vi "20190420 Subvi AO trigger old.vi"(9 "Delay_ticks":u32, 11 "Trigger":bool) -> (1 "IteratorDirection":bool, 3 "Stop":bool)   [LabVIEW 2017]
uses:
  GV trigger external AODO.vi
  GV frame counter.vi
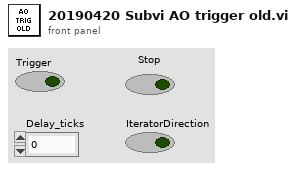
[diagram p1: front panel]
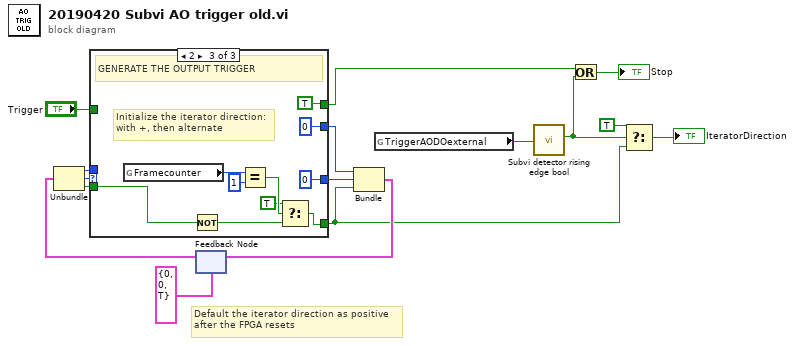
[diagram p0: block diagram]
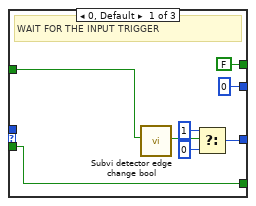
[diagram p2: hidden frame]
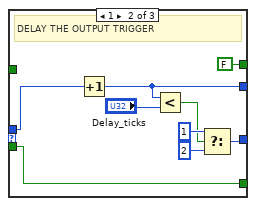
[diagram p3: hidden frame]
diagram:
  # "Default the iterator direction as positive\nafter the FPGA resets"
  n1 = feedback #1(cluster{u16, "f":u8, bool} {0, "f"=0, TRUE}) -> (w8:cluster{u32, "f":u8, bool})
  n2 = Unbundle(w8) -> (w9:u32, "f"=w11:u8, w12:bool)
  n3 = case shown="2" w11 {
    tunnel: [u32 0 w32 u32 0] -> w6
    tunnel: [w24 w28 u8 0 ("f")] -> w10
    tunnel: w9 -> [_ w33 _]
    tunnel: [FALSE FALSE TRUE] -> w2
    tunnel: [w19 w26 w34] -> w3
    tunnel: w12 -> [w19 w26 w36]
    tunnel: "Trigger" -> [w17 _ _]
    frame 0, Default {
      # "WAIT FOR THE INPUT TRIGGER"
      n4 = call "Subvi detector edge change bool.vi"("Input"=w17) -> ("Output"=w18:bool)  [unwired: 8 in]
      n5 = Select(t=u8 1, s=w18, f=u8 0) -> (s? t:f=w24:u8)
    }
    frame 1 {
      # "DELAY THE OUTPUT TRIGGER"
      n6 = Increment(x=w33) -> (x+1=w32:u32)
      n7 = Less?(x=w32, y="Delay_ticks") -> (x < y?=w30:bool)
      n8 = Select(t=u8 1, s=w30, f=u8 2) -> (s? t:f=w28:u8)
    }
    frame 2 {
      # "Initialize the iterator direction:\nwith +, then alternate"
      # "GENERATE THE OUTPUT TRIGGER"
      n9 = global read "GV frame counter.vi" "Framecounter"() -> (w38:i16)
      n10 = Not(x=w36) -> (.not. x?=w35:bool)
      n11 = Equal?(x=w38, y=i16 1) -> (x = y?=w40:bool)
      n12 = Select(t=TRUE, s=w40, f=w35) -> (s? t:f=w34:bool)
    }
  }
  n13 = Bundle(w6, "f"=w10, w3) -> (w7:cluster{u32, "f":u8, bool})  [unwired: 1 in]
  n14 = feedback-in #1(w7) -> ()
  n15 = global read "GV trigger external AODO.vi" "TriggerAODOexternal"() -> (w14:bool)
  n16 = call "Subvi detector rising edge bool.vi"("Input"=w14) -> ("Output"=w1:bool)  [unwired: 10 in]
  n17 = Or(x=w2, y=w1) -> (x .or. y?=→"Stop":bool)
  n18 = Select(t=TRUE, s=w1, f=w3) -> (s? t:f=→"IteratorDirection":bool)
